vi "Fail-Safe Control FPGA.vi"() -> ()   [LabVIEW 2017]
uses:
  Type Defs/Fail-Safe FPGA States.ctl
  <vilib>/rvi/Emulation/niFpgaSctlEmulationGetInTimedLoop.vi
  <vilib>/rvi/Emulation/niFpgaProcessEmulError.vi
  Storage/Fail-Safe Control FPGA Globals.vi
  <vilib>/rvi/Emulation/niFpgaGetClockAttributes.vi
  <vilib>/rvi/Emulation/niFpgaEmulationReportErrorSimple.vi
  <vilib>/rvi/eio/common/nirviEmuTemplateMethod_errors.vi
  <vilib>/rvi/Emulation/niFpgaCriticalErrorInLSC.vi
  <vilib>/eio/EIONode/EIONode.xnode
panel:
  in  "Digital Control Outputs":bool[](array[boolean])=[FALSE, FALSE, FALSE, FALSE, FALSE, FALSE, FALSE, FALSE, FALSE, FALSE, FALSE, FALSE, FALSE, FALSE, FALSE, FALSE]
  in  "Update Period (us)":u32=100000
  in  "RT Reset on Watchdog Failure?":bool
  in  "Enable RT Watchdog":bool
  in  "Pet RT Watchdog":bool
  in  "RT Timeout Period (ticks)":u32=40000000 format="%.0p"
  out "Time Since Last RT Pet":u32 format="%#.5p"
  in  "RT Safe":bool
  # "Configuration"
  # "Control Outputs From Host"
  # "Debug/RT Access"
  # "RT Flags"
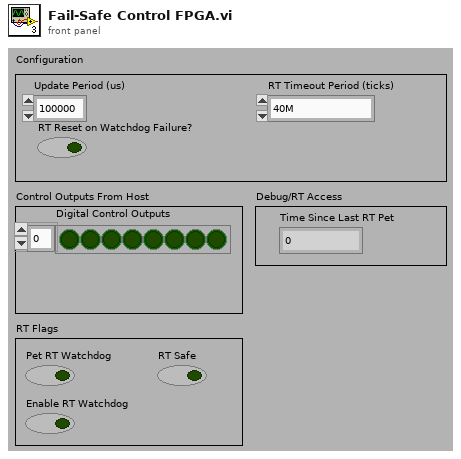
[diagram p1: front panel]
types:
  T1 = typedef "Fail-Safe FPGA States.ctl" = enum16{"Normal Operation", "Safe State"}
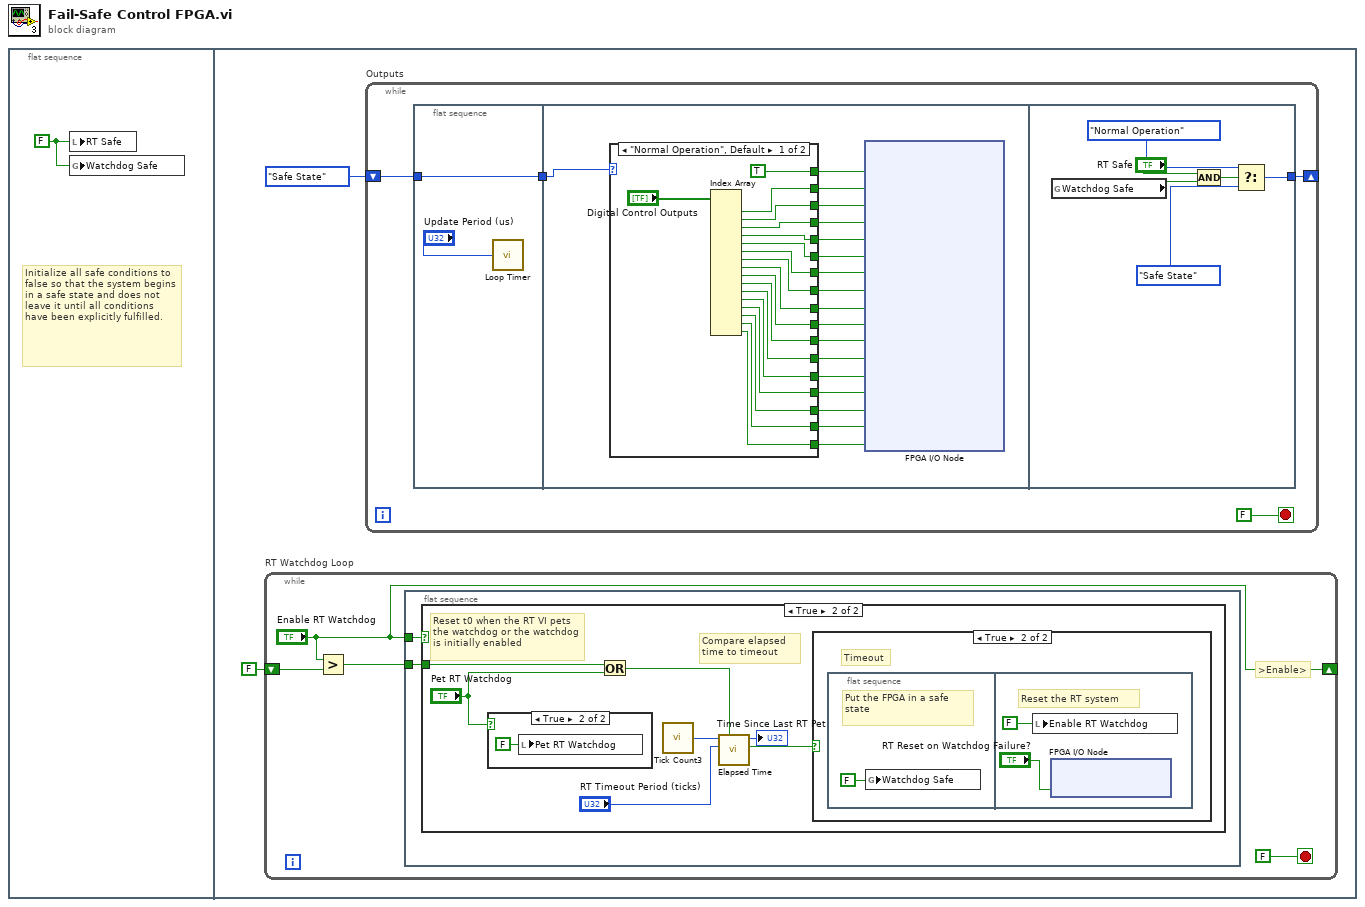
[diagram p0: block diagram]
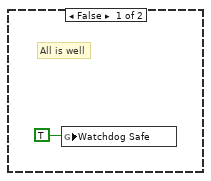
[diagram p3: hidden frame]
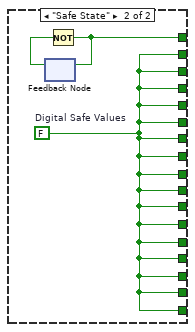
[diagram p5: hidden frame]
diagram:
  n1 = flat-sequence {
    frame #0 {
      w1 = FALSE ("RT Safe")
      # "Initialize all safe conditions to false so that the system begins in a safe state and does not leave it until all conditions have been explicitly fulfilled."
      n2 = local write "RT Safe"(w1) -> ()
      n3 = global write "Fail-Safe Control FPGA Globals.vi" "Watchdog Safe"(w1) -> ()
    }
    frame #1 {
      n4 = while "RT Watchdog Loop" {
        shift-right: ["Enable RT Watchdog"] -> _
        shift-left: FALSE ("Enable RT Watchdog 2") -> [w7]
        stop <- FALSE stop-if-true
        # ">Enable>"
        n5 = Greater?(x="Enable RT Watchdog", y=w7) -> (0:w4:bool)
        n6 = flat-sequence {
          tunnel: "Enable RT Watchdog" -> [w9]
          tunnel: w4 -> [w8]
          frame #0 {
            n7 = case shown="True" w9 {
              tunnel: w8 -> [_ w12]
              frame False {
                # "This loop has to be explicitly enabled from the RT program.  This reduces the possiblity of an endless reboot cycle."
              }
              frame True {
                # "Compare elapsed time to timeout"
                # "Reset t0 when the RT VI pets the watchdog or the watchdog is initially enabled"
                n8 = case shown="True" "Pet RT Watchdog" {
                  frame False {
                  }
                  frame True {
                    n9 = local write "Pet RT Watchdog"(FALSE ("Pet RT Watchdog")) -> ()
                  }
                }
                n10 = Or(x=w12, y="Pet RT Watchdog") -> (x .or. y?=w11:bool)
                n11 = call "Tick Count3"() -> ("Tick Count(Ticks)"=w15:u32)
                n12 = call "Elapsed Time.vi"("Reset"=w11, "Timeout Period"="RT Timeout Period (ticks)", "Current Time"=w15) -> ("Timeout"=w10:bool, "Elapsed Time"=→"Time Since Last RT Pet":u64)  [unwired: 7 in]
                n13 = case shown="True" w10 {
                  frame False {
                    # "All is well"
                    n14 = global write "Fail-Safe Control FPGA Globals.vi" "Watchdog Safe"(TRUE ("State Change")) -> ()
                  }
                  frame True {
                    # "Timeout"
                    n15 = flat-sequence {
                      frame #0 {
                        # "Put the FPGA in a safe\nstate"
                        n16 = global write "Fail-Safe Control FPGA Globals.vi" "Watchdog Safe"(FALSE ("State Change")) -> ()
                      }
                      frame #1 {
                        # "Reset the RT system"
                        n17 = local write "Enable RT Watchdog"(FALSE ("Enable RT Watchdog")) -> ()
                        n18 = xnode "FPGA I/O Node"("System Reset"="RT Reset on Watchdog Failure?") -> ()  [unwired: 1 in, 1 out]
                      }
                    }
                  }
                }
              }
            }
          }
        }
      }
      n19 = while "Outputs" {
        shift-right: [w23] -> _
        shift-left: Fail-Safe_FPGA_States."Safe State" ("State") -> [w24]
        stop <- FALSE stop-if-true
        n20 = flat-sequence {
          tunnel: w24 -> [w27]
          tunnel: [w27] -> w22
          tunnel: w22 -> [w45]
          tunnel: [w68] -> w23
          frame #0 {
            n21 = call "Loop Timer"("Count(uSec)"="Update Period (us)") -> ()  [unwired: 1 out]
          }
          frame #1 {
            n22 = case shown="\"Normal Operation\", Default" w45 {
              tunnel: [TRUE w65] -> w44
              tunnel: [w61 w64] -> w43
              tunnel: [w60 w64] -> w42
              tunnel: [w59 w64] -> w41
              tunnel: [w58 w64] -> w40
              tunnel: [w57 w64] -> w39
              tunnel: [w56 w64] -> w38
              tunnel: [w55 w64] -> w29
              tunnel: [w54 w64] -> w28
              tunnel: [w53 w64] -> w37
              tunnel: [w52 w64] -> w36
              tunnel: [w51 w64] -> w35
              tunnel: [w50 w64] -> w34
              tunnel: [w49 w64] -> w33
              tunnel: [w48 w64] -> w32
              tunnel: [w47 w64] -> w31
              tunnel: [w46 w64] -> w30
              frame "Normal Operation", Default {
                n23 = Index Array(array="Digital Control Outputs") -> (element #1=w61:bool, element #2=w60:bool, element #3=w59:bool, element #4=w58:bool, element #5=w57:bool, element #6=w56:bool, element #7=w55:bool, element #8=w54:bool, element #9=w53:bool, element #10=w52:bool, element #11=w51:bool, element #12=w50:bool, element #13=w49:bool, element #14=w48:bool, element #15=w47:bool, element #16=w46:bool)  [unwired: 16 in]
              }
              frame "Safe State" {
                w64 = FALSE  # Digital Safe Values
                n24 = feedback #1() -> (w66:bool)  [unwired: 1 in]
                n25 = Not(x=w66) -> (.not. x?=w65:bool)
                n26 = feedback-in #1(w65) -> ()
              }
            }
            n27 = xnode "FPGA I/O Node"("USER FPGA LED"=w44, "lowVDCRail"=w43, "dumpValve"=w42, "brakeDO"=w41, "clamp"=w40, "pump"=w39, "ignition"=w38, "DigitalOut1/DO6"=w29, "DigitalOut1/DO7"=w28, "highSide"=w37, "preCharge"=w36, "lowSide"=w35, "Mod3/DO3"=w34, "Mod3/DO4"=w33, "Mod3/DO5"=w32, "Mod3/DO6"=w31, "Mod3/DO7"=w30) -> ()  [unwired: 17 in, 17 out]
          }
          frame #2 {
            n28 = global read "Fail-Safe Control FPGA Globals.vi" "Watchdog Safe"() -> (w67:bool)
            n29 = Compound Arithmetic op=AND("RT Safe", w67) -> (w71:bool)
            n30 = Select(t=Fail-Safe_FPGA_States."Normal Operation", s=w71, f=Fail-Safe_FPGA_States."Safe State" ("State")) -> (s? t:f=w68:T1)
          }
        }
      }
    }
  }
